vi "Save XML.vi"(8 "Error In":errorcluster, 9 "Save UIP List (True)":bool=TRUE, 10 "UIM XML Path":path, 11 "UIM In":refnum<data-value>) -> (0 "Error Out":errorcluster, 3 "UIM Out":refnum<data-value>)   [LabVIEW 2020, in "UIM.lvlib" / "UIM.lvclass"]
doc: "Save the UI Manager data to an XML file. Setting the Save UIP List to True will add the UIPList entry to the XML file. This entry will be loaded when the file is loaded as the UIPs to be used."
uses:
  UIM.lvclass
  <vilib>/xml/Close Reference(Node).vi
  <vilib>/xml/NI_XML.lvlib
  <resource>/objmgr/DOMUserDefRef.rc
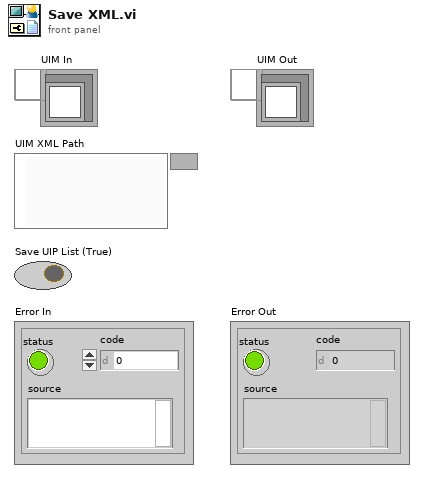
[diagram p1: front panel]
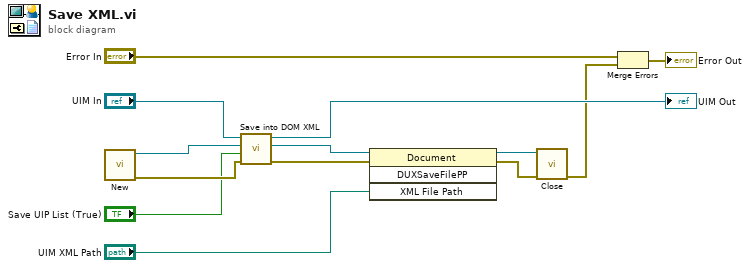
[diagram p0: block diagram]
diagram:
  n1 = call <vilib>:"New.vi"() -> ("error out"=w8:errorcluster, "DOM document out"=w7:refnum<k20>)  [unwired: 8 in]
  n2 = call "Save into DOM XML.vi"("Error In"=w8, "Save UIP List (True)"="Save UIP List (True)", "DOM In"=w7, "UIM In"="UIM In") -> ("Error Out"=w4:errorcluster, "DOM Out"=w3:refnum<k20>, "UIM Out"=→"UIM Out":refnum<data-value>)  [unwired: 5 in]
  n3 = invoke class="Document" method="DUXSaveFilePP"(reference=w3, error in=w4, "XML File Path"="UIM XML Path") -> (reference out=w11:refnum<k20>, error out=w10:errorcluster)  [unwired: 1 in, 2 out]
  n4 = call-poly <vilib>:"Close.vi"("error in (no error)"=w10, "node"=w11) -> ("error out"=w1:errorcluster)  [unwired: 7 in]
  n5 = Merge Errors("Error In", w1) -> (→"Error Out":errorcluster)
